vi "事件状态机.vi"() -> ()   [LabVIEW 2015]
uses:
  <vilib>/Utility/file.llb/Write Delimited Spreadsheet (DBL).vi
panel:
  in  "开始采集":bool
  in  "停止":bool
  out "波形图表":dbl(graph)
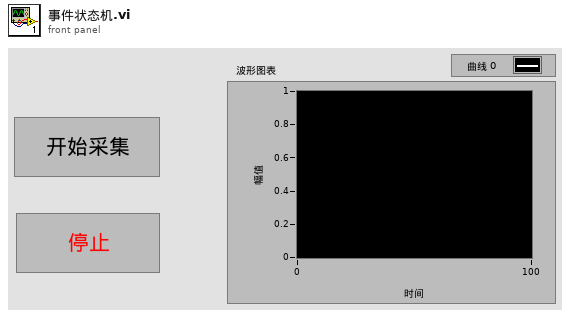
[diagram p1: front panel]
types:
  T1 = enum16{"open", "replace", "create", "open or create", "replace or create", "replace or create with confirmation"}
  T2 = cluster{"数据保存 Stop":refnum<user-event>, "数据显示 Stop":refnum<user-event>, "数据采集 Stop":refnum<user-event>, "操作面板 Stop":refnum<user-event>, "开始采集":refnum<user-event>, "保存数据":refnum<user-event>, "显示数据":refnum<user-event>}
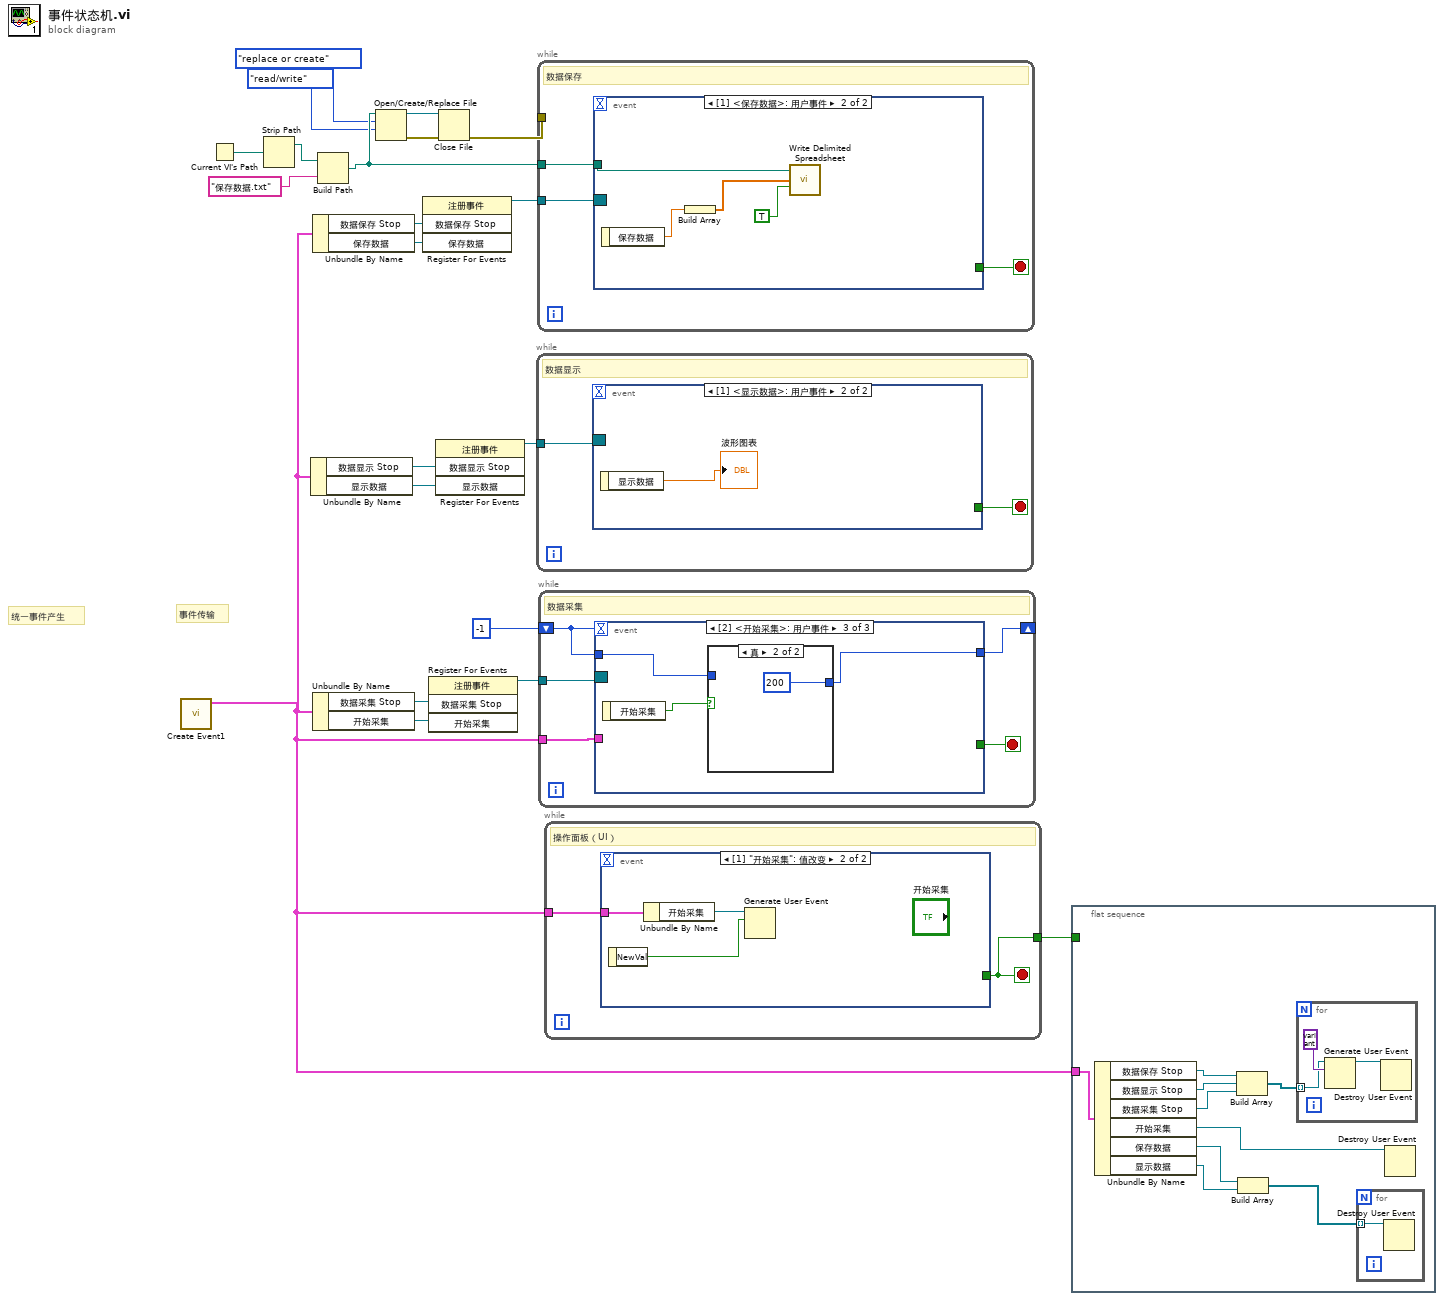
[diagram p0: block diagram]
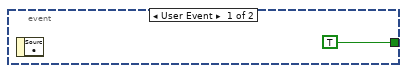
[diagram p2: hidden frame]
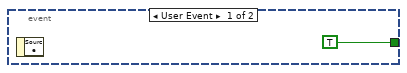
[diagram p3: hidden frame]
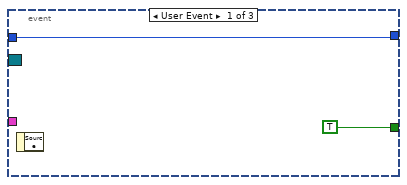
[diagram p4: hidden frame]
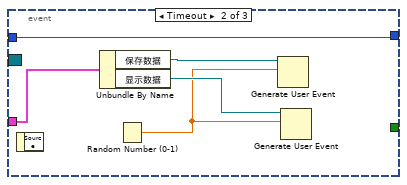
[diagram p5: hidden frame]
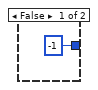
[diagram p6: hidden frame]
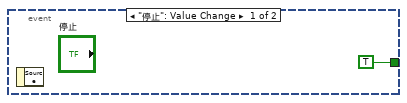
[diagram p7: hidden frame]
diagram:
  # "事件传输"
  # "统一事件产生"
  n1 = call "Create Event1.vi"() -> ("Event Out"=w12:T2)  [unwired: 11 in]
  n2 = Current VI's Path() -> (path=w10:path)
  n3 = Strip Path(path=w10) -> (stripped path=w9:path)  [unwired: 1 out]
  n4 = Unbundle By Name(w12) -> ("数据显示 Stop"=w18:refnum<user-event>, "显示数据"=w11:refnum<user-event>)
  n5 = Unbundle By Name(w12) -> ("数据保存 Stop"=w17:refnum<user-event>, "保存数据"=w7:refnum<user-event>)
  n6 = Unbundle By Name(w12) -> ("数据采集 Stop"=w16:refnum<user-event>, "开始采集"=w13:refnum<user-event>)
  n7 = Build Path(base path=w9, name or relative path="保存数据.txt" ("名称或相对路径")) -> (appended path=w6:path)
  n8 = Open/Create/Replace File(file path (use dialog)=w6, operation (0:open)=T1."replace or create" ("操作(0:open)"), access (0:read/write)=enum16{"read/write", "read-only", "write-only"}."read/write" ("权限(0:read/write)")) -> (refnum out=w2:refnum<file>, error out=w3:errorcluster)  [unwired: 3 in, 1 out]
  n9 = register-events(w17, w7) -> (reference out=w15:refnum<event-registration>)  [unwired: 2 in, 1 out]
  n10 = register-events(w16, w13) -> (reference out=w21:refnum<event-registration>)  [unwired: 2 in, 1 out]
  n11 = register-events(w18, w11) -> (reference out=w20:refnum<event-registration>)  [unwired: 2 in, 1 out]
  n12 = Close File(refnum=w2, error in=w3) -> (error out=w1:errorcluster)  [unwired: 1 out]
  n13 = while {
    tunnel: w20 -> [w23]
    stop <- w22 stop-if-true
    # "数据显示"
    n14 = event shown="[1] <显示数据>: 用户事件" {
      selector: w23 -> [_ _]
      dyn-events: _ -> [_ _]
      timeout: _ -> [_ _]
      tunnel: [TRUE _] -> w22
      event User Event {
        n15 = event-data() -> ()  [unwired: 1 in, 1 out]
      }
      event User Event {
        n16 = event-data() -> ("显示数据"=→"波形图表":dbl)  [unwired: 1 in]
      }
    }
  }
  n17 = while {
    tunnel: w15 -> [w27]
    tunnel: w6 -> [w26]
    tunnel: w1 -> [_]
    stop <- w28 stop-if-true
    # "数据保存"
    n18 = event shown="[1] <保存数据>: 用户事件" {
      selector: w27 -> [_ _]
      dyn-events: _ -> [_ _]
      timeout: _ -> [_ _]
      tunnel: [TRUE _] -> w28
      tunnel: w26 -> [_ w33]
      event User Event {
        n19 = event-data() -> ()  [unwired: 1 in, 1 out]
      }
      event User Event {
        n20 = event-data() -> ("保存数据"=w32:dbl)  [unwired: 1 in]
        n21 = Build Array(w32) -> (w31:dbl[])
        n22 = call-poly <vilib>:"Write Delimited Spreadsheet.vi"("file path (dialog if empty)"=w33, "1D data"=w31, "append to file? (F)"=TRUE) -> ()  [unwired: 11 in, 2 out]
      }
    }
  }
  n23 = while {
    tunnel: w21 -> [w38]
    shift-right: [w35] -> _
    shift-left: -1 -> [w36]
    tunnel: w12 -> [w34]
    stop <- w37 stop-if-true
    # "数据采集"
    n24 = event shown="[2] <开始采集>: 用户事件" {
      selector: w38 -> [_ _ _]
      dyn-events: _ -> [_ _ _]
      timeout: w36 -> [_ _ _]
      tunnel: [TRUE _ _] -> w37
      tunnel: [w39 w45 w46] -> w35
      tunnel: w36 -> [w39 w45 w47]
      tunnel: w34 -> [_ w44 _]
      event User Event {
        n25 = event-data() -> ()  [unwired: 1 in, 1 out]
      }
      event Timeout {
        n26 = event-data() -> ()  [unwired: 1 in, 1 out]
        n27 = Unbundle By Name(w44) -> ("保存数据"=w43:refnum<user-event>, "显示数据"=w42:refnum<user-event>)
        n28 = Random Number (0-1)() -> (number: 0 to 1=w41:dbl)
        n29 = Generate User Event(user event=w43, event data cluster=w41) -> ()  [unwired: 2 in, 2 out]
        n30 = Generate User Event(user event=w42, event data cluster=w41) -> ()  [unwired: 2 in, 2 out]
      }
      event User Event {
        n31 = event-data() -> ("开始采集"=w48:bool)  [unwired: 1 in]
        n32 = case shown="真" w48 {
          tunnel: w47 -> [_ _]
          tunnel: [-1 200] -> w46
          frame False {
          }
          frame True {
          }
        }
      }
    }
  }
  n33 = while {
    tunnel: [w52] -> w19
    tunnel: w12 -> [w51]
    stop <- w52 stop-if-true
    # "操作面板（UI）"
    n34 = event shown="[1] \"开始采集\": 值改变" {
      selector: _ -> [_ _]
      dyn-events: _ -> [_ _]
      timeout: _ -> [_ _]
      tunnel: [TRUE _] -> w52
      tunnel: w51 -> [_ w56]
      event "停止": Value Change {
        n35 = event-data() -> ()  [unwired: 1 in, 1 out]
      }
      event "开始采集": Value Change {
        n36 = event-data() -> ("NewVal"=w54:bool)  [unwired: 1 in]
        n37 = Unbundle By Name(w56) -> ("开始采集"=w55:refnum<user-event>)
        n38 = Generate User Event(user event=w55, event data cluster=w54) -> ()  [unwired: 2 in, 2 out]
      }
    }
  }
  n39 = flat-sequence {
    tunnel: w19 -> [_]
    tunnel: w12 -> [w65]
    frame #0 {
      n40 = Unbundle By Name(w65) -> ("数据保存 Stop"=w64:refnum<user-event>, "数据显示 Stop"=w63:refnum<user-event>, "数据采集 Stop"=w62:refnum<user-event>, "开始采集"=w60:refnum<user-event>, "保存数据"=w59:refnum<user-event>, "显示数据"=w58:refnum<user-event>)
      n41 = Build Array(w64, w63, w62) -> (w61:refnum<user-event>[])
      n42 = Build Array(w59, w58) -> (w57:refnum<user-event>[])
      n43 = for {
        tunnel: w61 -> [w67] mode=indexing
        n44 = Generate User Event(user event=w67, event data cluster=variant ("事件数据")) -> (user event out=w69:refnum<user-event>)  [unwired: 2 in, 1 out]
        n45 = Destroy User Event(user event=w69) -> ()  [unwired: 1 in, 1 out]
      }
      n46 = for {
        tunnel: w57 -> [w66] mode=indexing
        n47 = Destroy User Event(user event=w66) -> ()  [unwired: 1 in, 1 out]
      }
      n48 = Destroy User Event(user event=w60) -> ()  [unwired: 1 in, 1 out]
    }
  }
